vi "2013_01_05 Durability8 Main.vi"() -> ()   [LabVIEW 2011]
uses:
  MotorTypeDef.ctl
  <vilib>/DAQmx/write.llb/DAQmx Write (Counter Time 1Chan 1Samp).vi
  <vilib>/DAQmx/read.llb/DAQmx Read (Analog 1D Wfm NChan NSamp).vi
  <vilib>/Utility/TradDaqScaling.llb/Convert Thermistor Reading (waveform).vi
  <vilib>/DAQmx/miscellaneous.llb/DAQmx Fill In Error Info.vi
panel:
  in  "Y axis":u16(ring)=3 items=["RMS Current (A) 1"=1, "RMS Voltage (V) 1"=2, "RPM"=3, "Supply (V)"=4, "Torque (mNm)"=5, "Electrical Power (W)"=6, "Mechanical Power(W)"=7, "Motor Efficiency (%)"=8, "Source Current (A)"=10, "Supply Power (W)"=11, "ESC Efficiency (%)"=12, "Flow"=13, "Pressure Blue"=14, "Pressure Yellow"=15, "etc"=16]
  in  "X axis":u16(ring) items=["RMS Current (A) 1"=1, "RMS Voltage (V) 1"=2, "RPM"=3, "Supply (V)"=4, "Torque (mNm)"=5, "Electrical Power (W)"=6, "Mechanical Power(W)"=7, "Motor Efficiency (%)"=8, "Source Current (A)"=10, "Supply Power (W)"=11, "ESC Efficiency (%)"=12, "Flow"=13, "Pressure Blue"=14, "Pressure Yellow"=15, "Elapsed Time (s)"=0]
  out "XY Graph 2":cluster{"Array":dbl[], "Array":dbl[]}[](graph)
  out "Single Motor 2":waveform(dbl)[](graph)
  in  "Waveform":bool
  in  "Motor":dbl=1.0 min=1.0 max=8.0 step=1.0
  out "XY Graph":cluster{"Array":dbl[], "Array":dbl[]}[](graph)
  out "error out":errorcluster
  in  "File Path":path=path "Durability/.lvm"
  in  "Motor 8":T1 {"Power Input (W)" format="%.3g"; "Efficiency" format="%#_3g%%"; "Power Output (W)" format="%.3g"; "Torque (mNm)" format="%.3g"; "Elapsed Time" format="%<%H:%M:%S>t"; "Supply (V)" format="%.2f"; "RPM" scale=0.0..40000.0 scale format="%#_4p"}
  in  "Motor 7":T1 {"Power Input (W)" format="%.3g"; "Efficiency" format="%#_3g%%"; "Power Output (W)" format="%.3g"; "Torque (mNm)" format="%.3g"; "Elapsed Time" format="%<%H:%M:%S>t"; "Supply (V)" format="%.2f"; "RPM" scale=0.0..40000.0 scale format="%#_4p"}
  in  "Motor 6":T1 {"Power Input (W)" format="%.3g"; "Efficiency" format="%#_3g%%"; "Power Output (W)" format="%.3g"; "Torque (mNm)" format="%.3g"; "Elapsed Time" format="%<%H:%M:%S>t"; "Supply (V)" format="%.2f"; "RPM" scale=0.0..40000.0 scale format="%#_4p"}
  in  "Motor 5":T1 {"Power Input (W)" format="%.3g"; "Efficiency" format="%#_3g%%"; "Power Output (W)" format="%.3g"; "Torque (mNm)" format="%.3g"; "Elapsed Time" format="%<%H:%M:%S>t"; "Supply (V)" format="%.2f"; "RPM" scale=0.0..40000.0 scale format="%#_4p"}
  in  "Motor 4":T1 {"Power Input (W)" format="%.3g"; "Efficiency" format="%#_3g%%"; "Power Output (W)" format="%.3g"; "Torque (mNm)" format="%.3g"; "Elapsed Time" format="%<%H:%M:%S>t"; "Supply (V)" format="%.2f"; "RPM" scale=0.0..40000.0 scale format="%#_4p"}
  in  "Motor 3":T1 {"Power Input (W)" format="%.3g"; "Efficiency" format="%#_3g%%"; "Power Output (W)" format="%.3g"; "Torque (mNm)" format="%.3g"; "Elapsed Time" format="%<%H:%M:%S>t"; "Supply (V)" format="%.2f"; "RPM" scale=0.0..40000.0 scale format="%#_4p"}
  in  "Motor 2":T1 {"Power Input (W)" format="%.3g"; "Efficiency" format="%#_3g%%"; "Power Output (W)" format="%.3g"; "Torque (mNm)" format="%.3g"; "Elapsed Time" format="%<%H:%M:%S>t"; "Supply (V)" format="%.2f"; "RPM" scale=0.0..40000.0 scale format="%#_4p"}
  in  "Motor 1":T1 {"Power Input (W)" format="%.3g"; "Efficiency" format="%#_3g%%"; "Power Output (W)" format="%.3g"; "Torque (mNm)" format="%.3g"; "Elapsed Time" format="%<%H:%M:%S>t"; "Supply (V)" format="%.2f"; "RPM" scale=0.0..40000.0 scale format="%#_4p"}
  out "Motor Temp":dbl(slide) scale=65.0..110.0
  out "Tank Temp":dbl(slide) scale=65.0..110.0
  in  "Temp Probe\nOn Motor":dbl=1.0
  out "loop time (ms)":u32
  in  "stop":bool
  in  "Unlock PWM":bool=TRUE
  in  "PWM 2":dbl(slide)=100.0 min=0.0 max=100.0 step=5.0 scale=0.0..100.0
  in  "PWM 1":dbl(slide) min=0.0 max=100.0 step=5.0 scale=0.0..100.0
  # "Enable"
  # "Fail"
  # "Enable"
  # "Fail"
  # "Enable"
  # "Fail"
  # "Enable"
  # "Fail"
  # "Enable"
  # "Fail"
  # "Enable"
  # "Fail"
  # "Enable"
  # "Fail"
  # "Enable"
  # "Fail"
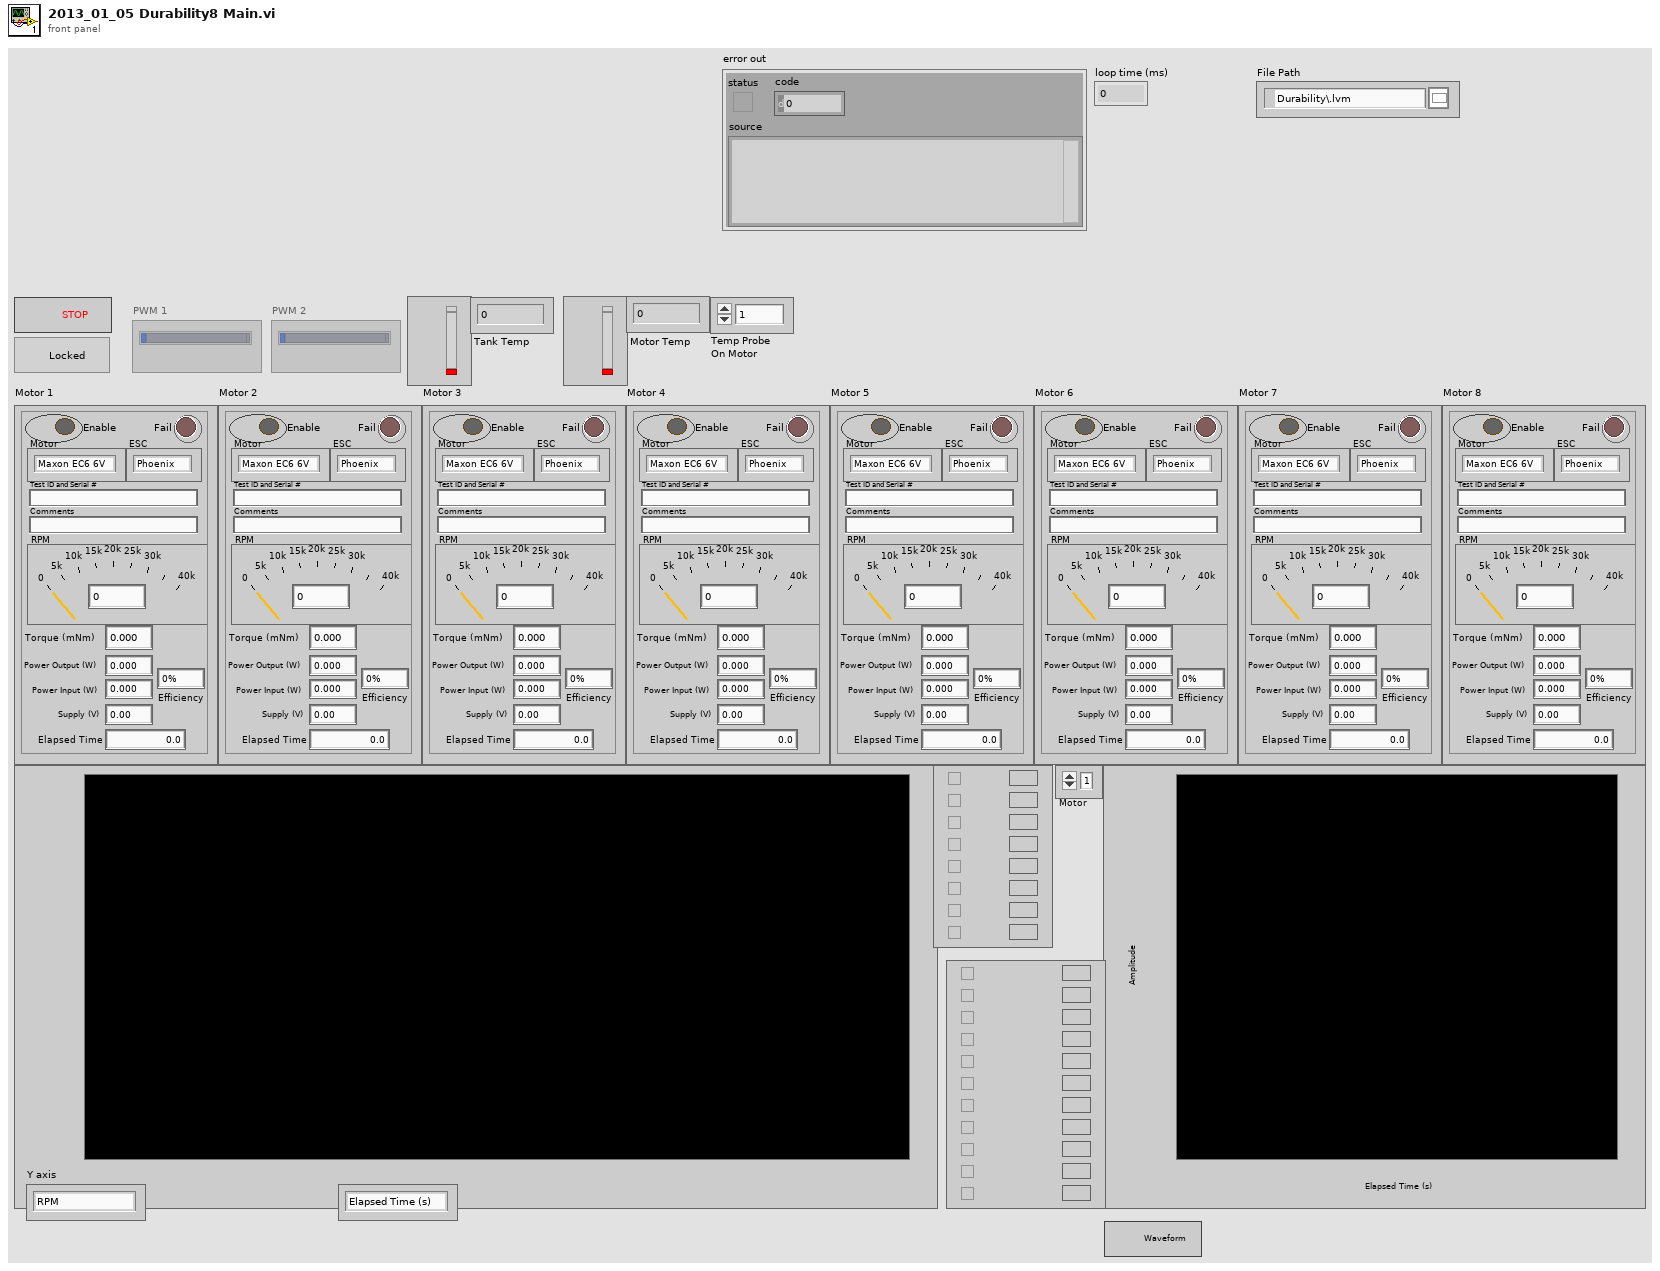
[diagram p1: front panel]
types:
  T1 = typedef "MotorTypeDef.ctl" = cluster{"Enabled":bool, "Fail":bool, "RPM":dbl, "Motor":enum16{"Maxon EC6 6V", "Maxon EC4 6V", "FH 0620 6V", "FH 0620 12V"}, "ESC":enum16{"Phoenix", "Maxon", "FH 1801"}, "Supply (V)":dbl, "Test ID and Serial #":string, "Comments":string, "Elapsed Time":dbl, "Counter":dbl, "Torque (mNm)":dbl, "Power Output (W)":dbl, "Efficiency":dbl, "Power Input (W)":dbl}
  T2 = enum8{"Enabled", "Disabled", "Disabled and Grayed Out"}
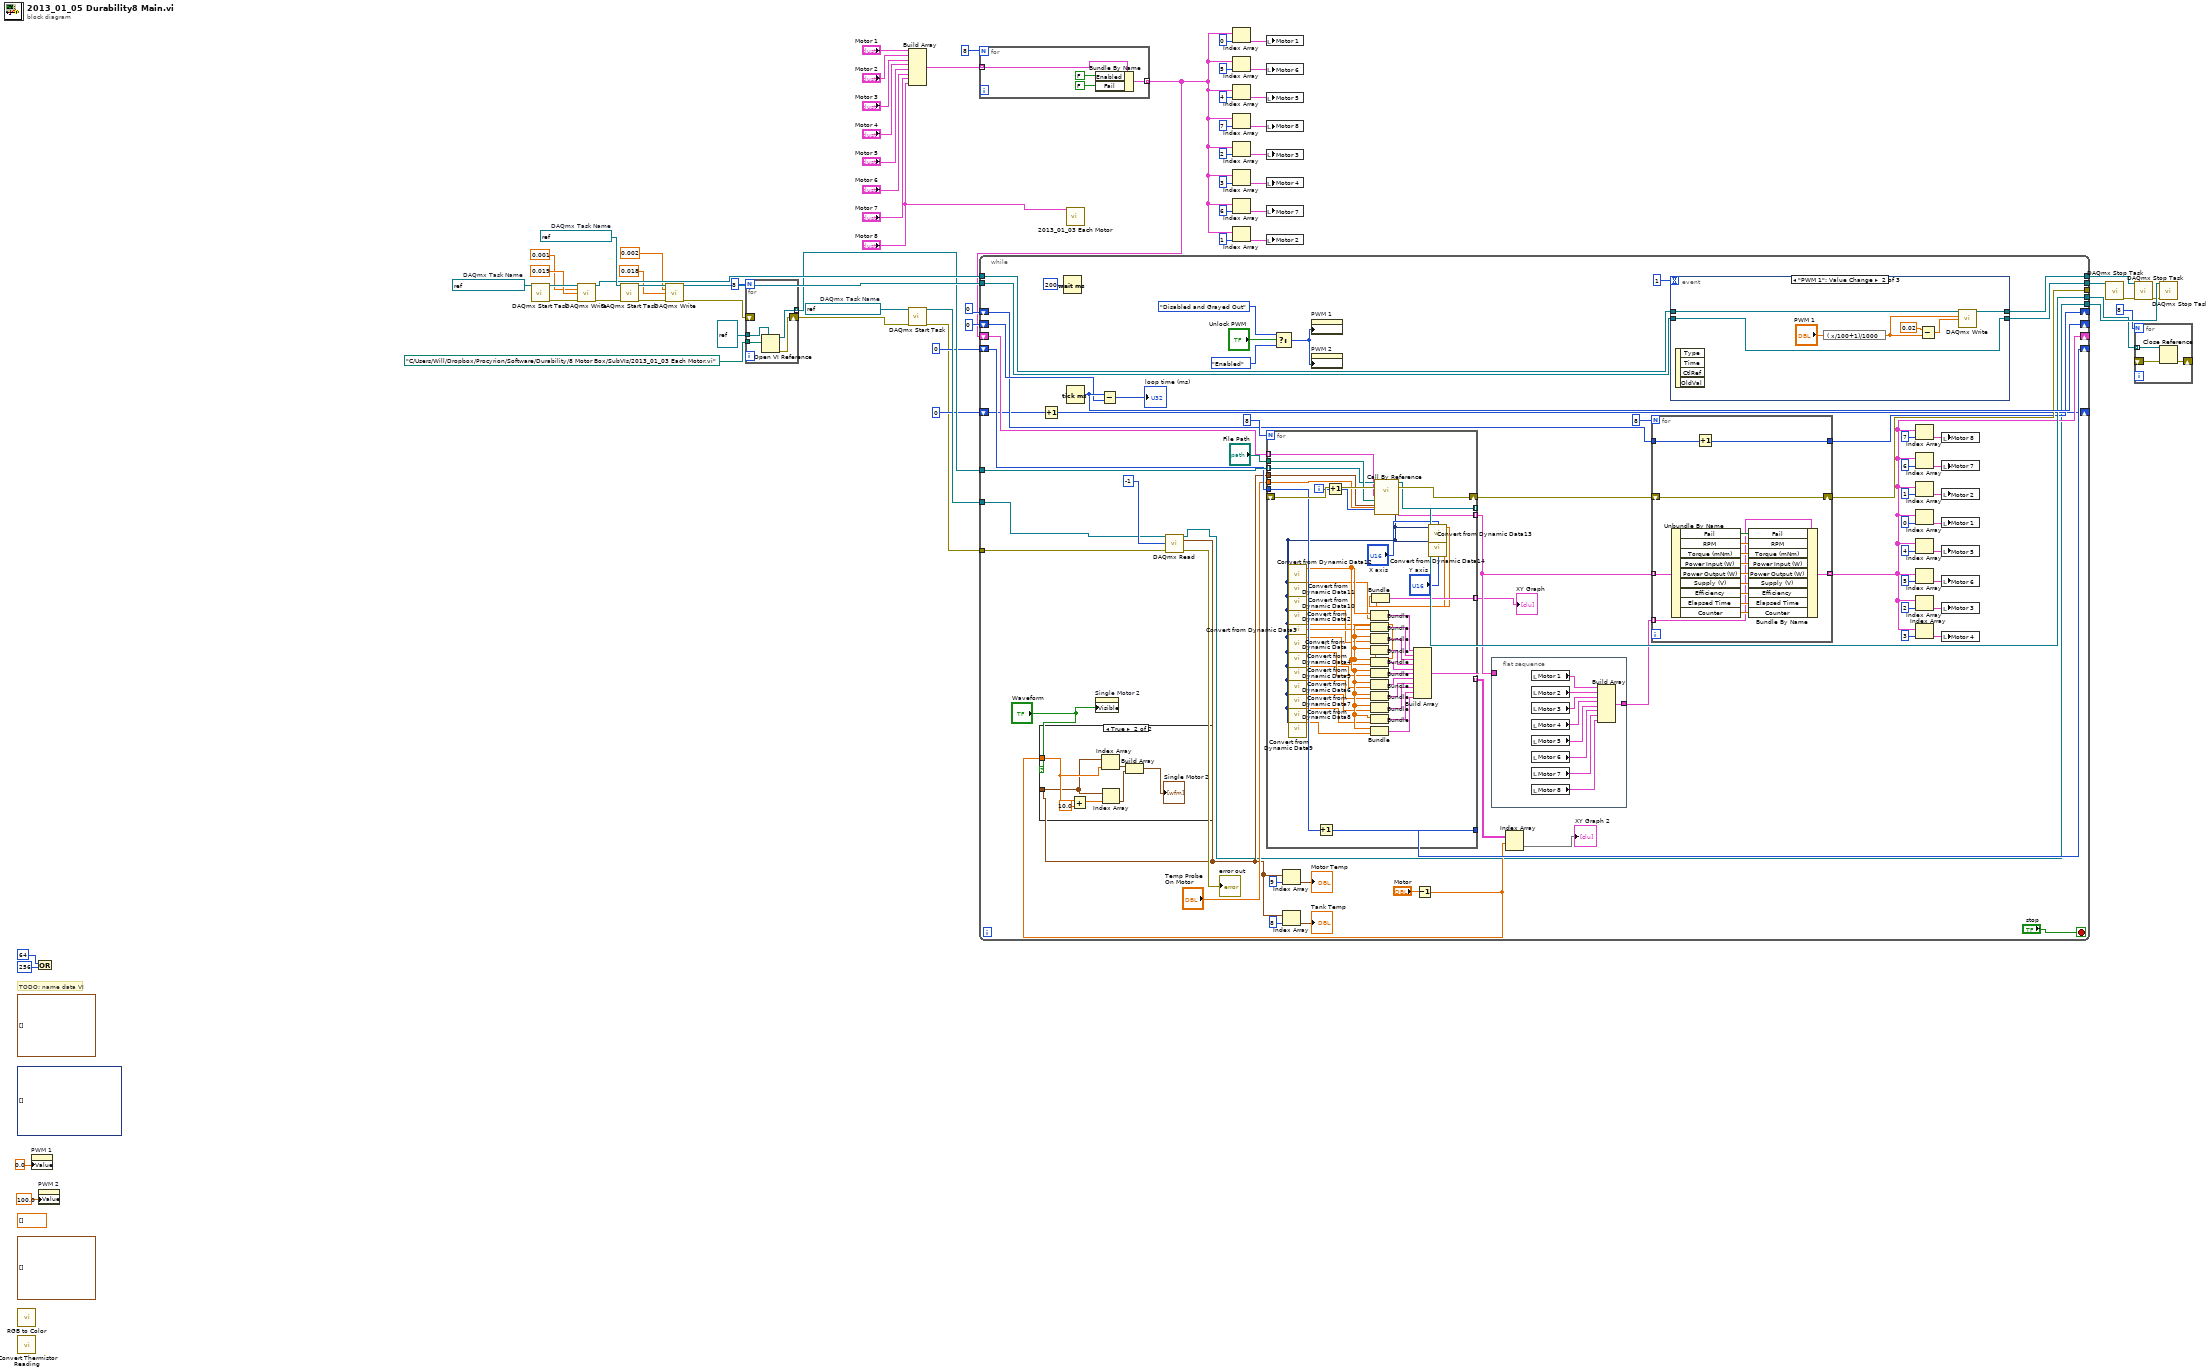
[diagram p0: block diagram]
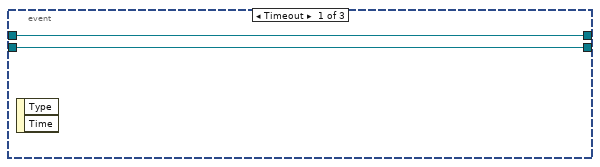
[diagram p3: hidden frame]
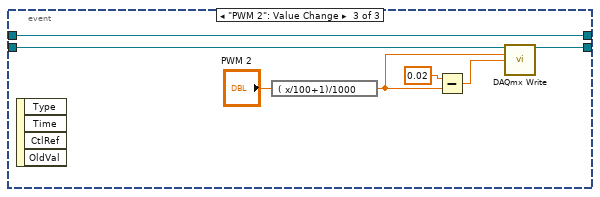
[diagram p4: hidden frame]
diagram:
  (unwired) dynamicdata[] []
  (unwired) dbl[] [] ("History Data")
  (unwired) waveform(dbl)[][] [] ("History Data")
  (unwired) waveform(dbl)[][] [] ("History Data")
  w60 = refnum<k21> "Durability8 PWM2"  # DAQmx Task Name
  w61 = refnum<k21> "Durability8 PWM1"  # DAQmx Task Name
  w64 = refnum<k21> "Durability8 Acquire"  # DAQmx Task Name
  # "TODO: name data VI"
  n1 = call <vilib>:"RGB to Color.vi"() -> ()  [unwired: 3 in, 1 out]
  n2 = call-poly <vilib>:"Convert Thermistor Reading.vi"() -> ()  [unwired: 7 in, 1 out]
  n3 = property on="PWM 1" class="Slide (strict)"("Value"=0.0 ("PWM 1")) -> ()  [unwired: 2 in, 2 out]
  n4 = Compound Arithmetic op=OR(64 ("options"), 256 ("options")) -> ()  [unwired: 1 out]
  n5 = property on="PWM 2" class="Slide (strict)"("Value"=100.0 ("PWM 2")) -> ()  [unwired: 2 in, 2 out]
  n6 = call <vilib>:"DAQmx Start Task.vi"("task/channels in"=w61) -> ("task out"=w57:refnum<k21>, "error out"=w55:errorcluster)  [unwired: 13 in]
  n7 = call-poly <vilib>:"DAQmx Write.vi"("task/channels in"=w57, "high time"=0.001 ("data"), "low time"=0.019 ("data"), "error in"=w55) -> ("task out"=w59:refnum<k21>, "error out"=w54:errorcluster)  [unwired: 9 in, 1 out]
  n8 = call <vilib>:"DAQmx Start Task.vi"("task/channels in"=w60, "error in"=w54) -> ("task out"=w56:refnum<k21>, "error out"=w53:errorcluster)  [unwired: 12 in]
  n9 = call-poly <vilib>:"DAQmx Write.vi"("task/channels in"=w56, "high time"=0.002 ("data"), "low time"=0.018 ("data"), "error in"=w53) -> ("task out"=w58:refnum<k21>, "error out"=w22:errorcluster)  [unwired: 9 in, 1 out]
  n10 = for {
    N: 8 -> [_]
    tunnel: path "C:/Users/Will/Dropbox/Procyrion/Software/Durability/8 Motor Box/SubVIs/2013_01_03 Each Motor.vi" -> [w68]
    tunnel: [w67] -> w38 mode=indexing
    tunnel: refnum<vi> refnum ("type specifier VI Refnum (for type only)") -> [w66]
    shift-right: [w65] -> w23
    shift-left: w22 -> [_]
    n11 = Open VI Reference(type specifier VI Refnum (for type only)=w66, vi path=w68) -> (vi reference=w67:refnum<vi>, error out=w65:errorcluster)  [unwired: 4 in]
  }
  n12 = Build Array("Motor 1", "Motor 2", "Motor 3", "Motor 4", "Motor 5", "Motor 6", "Motor 7", "Motor 8") -> (w19:T1[])
  n13 = call <vilib>:"DAQmx Start Task.vi"("task/channels in"=w64, "error in"=w23) -> ("task out"=w63:refnum<k21>, "error out"=w21:errorcluster)  [unwired: 12 in]
  n14 = for {
    N: 8 -> [_]
    tunnel: w19 -> [w72] mode=indexing
    tunnel: [w69] -> w2 mode=indexing
    n15 = Bundle By Name(cluster=w72, "Enabled"=FALSE, "Fail"=FALSE) -> (w69:T1)
  }
  n16 = while {
    tunnel: w63 -> [w73]
    tunnel: [w76] -> w62
    tunnel: w21 -> [w96]
    shift-right: [w132] -> _
    shift-left: u32 0 ("millisecond timer value") -> [w131]
    tunnel: w59 -> [w124]
    tunnel: w58 -> [w123]
    tunnel: [w122] -> w52
    tunnel: [w121] -> w45
    tunnel: w38 -> [w117]
    tunnel: [w116] -> w34
    shift-right: [w98] -> _
    shift-left: w2 -> [w97]
    tunnel: [w95] -> _
    shift-right: [w92] -> _
    shift-left: 0 ("for") -> [w93]
    shift-right: [w90] -> _
    shift-left: 0 ("for") -> [w91]
    shift-right: [w88] -> _
    shift-left: 0 ("for") -> [w89]
    stop <- "stop" stop-if-true
    n17 = Increment(x=w89) -> (x+1=w88:i32)
    n18 = Wait (ms)(milliseconds to wait=u32 200) -> ()  [unwired: 1 out]
    n19 = Tick Count (ms)() -> (millisecond timer value=w132:u32)
    n20 = property on="Single Motor 2" class="WFGraph (strict)"("Visible"="Waveform") -> ()  [unwired: 2 in, 2 out]
    n21 = Subtract(x=w132, y=w131) -> (x-y=→"loop time (ms)":u32)
    n22 = call-poly <vilib>:"DAQmx Read.vi"("task/channels in"=w73, "number of samples per channel"=-1, "error in"=w96) -> ("task out"=w76:refnum<k21>, "data"=w79:waveform(dbl)[], "error out"=→"error out":errorcluster)  [unwired: 10 in]
    n23 = for {
      N: 8 -> [_]
      tunnel: w79 -> [w222]
      tunnel: "File Path" -> [w223]
      tunnel: w117 -> [w220] mode=indexing
      shift-right: [w226] -> w94
      shift-left: _ -> [w225]
      tunnel: [w219] -> w116 mode=indexing
      tunnel: [w218] -> w86 mode=indexing
      tunnel: w97 -> [w184] mode=indexing
      tunnel: w93 -> [w217]
      tunnel: [w216] -> w92
      tunnel: "Temp Probe\nOn Motor" -> [w215]
      tunnel: [w214] -> w81 mode=indexing
      tunnel: [w201] -> w75 mode=indexing
      i -> [w224]
      n24 = Increment(x=w217) -> (x+1=w216:i32)
      n25 = Increment(x=w224) -> (x+1=w221:i32)
      n26 = call-by-ref "?"(reference=w220, error in=w225, "Temp On"=w215, "Motor #"=w221, "data"=w222, "File Path"=w223, "Motor Typedef"=w184) -> (reference out=w219:refnum<vi>, error out=w226:errorcluster, "Final Out"=w187:dynamicdata, "Motor Typedef Out"=w218:T1)  [unwired: 5 in]
      n27 = call "Convert from Dynamic Data12"("Dynamic Data Type"=w187) -> ("Array"=w202:dbl[])  [unwired: 3 in]
      n28 = call "Convert from Dynamic Data11"("Dynamic Data Type"=w187) -> ("Array"=w200:dbl[])  [unwired: 3 in]
      n29 = call "Convert from Dynamic Data10"("Dynamic Data Type"=w187) -> ("Array"=w199:dbl[])  [unwired: 3 in]
      n30 = call "Convert from Dynamic Data2"("Dynamic Data Type"=w187) -> ("Array"=w198:dbl[])  [unwired: 3 in]
      n31 = call "Convert from Dynamic Data3"("Dynamic Data Type"=w187) -> ("Array"=w197:dbl[])  [unwired: 3 in]
      n32 = call "Convert from Dynamic Data"("Dynamic Data Type"=w187) -> ("Array"=w196:dbl[])  [unwired: 3 in]
      n33 = call "Convert from Dynamic Data4"("Dynamic Data Type"=w187) -> ("Array"=w195:dbl[])  [unwired: 3 in]
      n34 = call "Convert from Dynamic Data5"("Dynamic Data Type"=w187) -> ("Array"=w194:dbl[])  [unwired: 3 in]
      n35 = call "Convert from Dynamic Data6"("Dynamic Data Type"=w187) -> ("Array"=w193:dbl[])  [unwired: 3 in]
      n36 = call "Convert from Dynamic Data7"("Dynamic Data Type"=w187) -> ("Array"=w192:dbl[])  [unwired: 3 in]
      n37 = call "Convert from Dynamic Data8"("Dynamic Data Type"=w187) -> ("Array"=w191:dbl[])  [unwired: 3 in]
      n38 = call "Convert from Dynamic Data9"("Dynamic Data Type"=w187) -> ("Array"=w190:dbl[])  [unwired: 3 in]
      n39 = Bundle("Array"=w202, "Array"=w200) -> (w203:cluster{"Array":dbl[], "Array":dbl[]})  [unwired: 1 in]
      n40 = Bundle("Array"=w202, "Array"=w199) -> (w204:cluster{"Array":dbl[], "Array":dbl[]})  [unwired: 1 in]
      n41 = Bundle("Array"=w202, "Array"=w198) -> (w205:cluster{"Array":dbl[], "Array":dbl[]})  [unwired: 1 in]
      n42 = Bundle("Array"=w202, "Array"=w197) -> (w206:cluster{"Array":dbl[], "Array":dbl[]})  [unwired: 1 in]
      n43 = Bundle("Array"=w202, "Array"=w196) -> (w207:cluster{"Array":dbl[], "Array":dbl[]})  [unwired: 1 in]
      n44 = Bundle("Array"=w202, "Array"=w195) -> (w208:cluster{"Array":dbl[], "Array":dbl[]})  [unwired: 1 in]
      n45 = Bundle("Array"=w202, "Array"=w194) -> (w209:cluster{"Array":dbl[], "Array":dbl[]})  [unwired: 1 in]
      n46 = Bundle("Array"=w202, "Array"=w193) -> (w210:cluster{"Array":dbl[], "Array":dbl[]})  [unwired: 1 in]
      n47 = Bundle("Array"=w202, "Array"=w192) -> (w212:cluster{"Array":dbl[], "Array":dbl[]})  [unwired: 1 in]
      n48 = Bundle("Array"=w202, "Array"=w191) -> (w211:cluster{"Array":dbl[], "Array":dbl[]})  [unwired: 1 in]
      n49 = Bundle("Array"=w202, "Array"=w190) -> (w213:cluster{"Array":dbl[], "Array":dbl[]})  [unwired: 1 in]
      n50 = Build Array(w203, w204, w205, w206, w207, w208, w209, w210, w212, w211, w213) -> (w201:cluster{"Array":dbl[], "Array":dbl[]}[])
      n51 = call "Convert from Dynamic Data13"("Dynamic Data Type"=w187, "Channel"="X axis") -> ("Array"=w186:dbl[])  [unwired: 2 in]
      n52 = call "Convert from Dynamic Data14"("Dynamic Data Type"=w187, "Channel"="Y axis") -> ("Array"=w185:dbl[])  [unwired: 2 in]
      n53 = Bundle("Array"=w186, "Array"=w185) -> (w214:cluster{"Array":dbl[], "Array":dbl[]})  [unwired: 1 in]
    }
    "XY Graph" <- w81
    n54 = Select(t=T2."Disabled and Grayed Out" ("Disabled"), s="Unlock PWM", f=T2."Enabled" ("Disabled")) -> (s? t:f=w136:T2)
    n55 = Index Array(array=w79, index=9) -> (element=→"Motor Temp":waveform(dbl))
    n56 = Index Array(array=w79, index=8) -> (element=→"Tank Temp":waveform(dbl))
    n57 = property on="PWM 1" class="Slide (strict)"("DisabledEnum"=w136) -> ()  [unwired: 2 in, 2 out]
    n58 = property on="PWM 2" class="Slide (strict)"("DisabledEnum"=w136) -> ()  [unwired: 2 in, 2 out]
    n59 = Decrement(x="Motor") -> (x-1=w78:dbl)
    n60 = case shown="True" "Waveform" {
      tunnel: w79 -> [_ w141]
      tunnel: w78 -> [_ w142]
      frame False {
      }
      frame True {
        n61 = Add(x=w142, y=10.0) -> (x+y=w140:dbl)
        n62 = Index Array(array=w141, index=w142) -> (element=w139:waveform(dbl))
        n63 = Index Array(array=w141, index=w140) -> (element=w138:waveform(dbl))
        n64 = Build Array(w139, w138) -> (→"Single Motor 2":waveform(dbl)[])
      }
    }
    n65 = flat-sequence {
      tunnel: [w145] -> w87
      tunnel: w86 -> [_]
      frame #0 {
        n66 = local read "Motor 1"() -> (w146:T1)
        n67 = local read "Motor 2"() -> (w147:T1)
        n68 = local read "Motor 3"() -> (w148:T1)
        n69 = local read "Motor 4"() -> (w149:T1)
        n70 = local read "Motor 5"() -> (w150:T1)
        n71 = local read "Motor 6"() -> (w151:T1)
        n72 = local read "Motor 7"() -> (w152:T1)
        n73 = local read "Motor 8"() -> (w144:T1)
        n74 = Build Array(w146, w147, w148, w149, w150, w151, w152, w144) -> (w145:T1[])
      }
    }
    n75 = Index Array(array=w75, index (row)=w78) -> (element=→"XY Graph 2":cluster{"Array":dbl[], "Array":dbl[]}[])  [unwired: 1 in]
    n76 = for {
      N: 8 -> [_]
      tunnel: w87 -> [w158] mode=indexing
      tunnel: [w157] -> w98 mode=indexing
      tunnel: w86 -> [w156] mode=indexing
      shift-right: [w155] -> w95
      shift-left: w94 -> [w155]
      tunnel: [w153] -> w90
      tunnel: w91 -> [w154]
      n77 = Unbundle By Name(w156) -> ("Fail"=w167:bool, "RPM"=w166:dbl, "Torque (mNm)"=w165:dbl, "Power Input (W)"=w164:dbl, "Power Output (W)"=w163:dbl, "Supply (V)"=w162:dbl, "Efficiency"=w161:dbl, "Elapsed Time"=w160:dbl, "Counter"=w159:dbl)
      n78 = Increment(x=w154) -> (x+1=w153:i32)
      n79 = Bundle By Name(cluster=w158, "Fail"=w167, "RPM"=w166, "Torque (mNm)"=w165, "Power Input (W)"=w164, "Power Output (W)"=w163, "Supply (V)"=w162, "Efficiency"=w161, "Elapsed Time"=w160, "Counter"=w159) -> (w157:T1)
    }
    n80 = event shown="[1] \"PWM 1\": Value Change" {
      selector: _ -> [_ _ _]
      dyn-events: _ -> [_ _ _]
      timeout: 1 -> [_ _ _]
      tunnel: w124 -> [w169 w172 w178]
      tunnel: w123 -> [w168 w170 w177]
      tunnel: [w169 w171 w178] -> w122
      tunnel: [w168 w170 w179] -> w121
      event Timeout {
        n81 = event-data() -> ()  [unwired: 1 in, 2 out]
      }
      event "PWM 1": Value Change {
        n82 = event-data() -> ()  [unwired: 1 in, 4 out]
        n83 = expression code="( x/100+1)/1000"("PWM 1") -> (w173:dbl)
        n84 = Subtract(x=0.02 ("y"), y=w173) -> (x-y=w174:dbl)
        n85 = call-poly <vilib>:"DAQmx Write.vi"("task/channels in"=w172, "high time"=w173, "low time"=w174) -> ("task out"=w171:refnum<k21>)  [unwired: 10 in, 2 out]
      }
      event "PWM 2": Value Change {
        n86 = event-data() -> ()  [unwired: 1 in, 4 out]
        n87 = expression code="( x/100+1)/1000"("PWM 2") -> (w183:dbl)
        n88 = Subtract(x=0.02, y=w183) -> (x-y=w181:dbl)
        n89 = call-poly <vilib>:"DAQmx Write.vi"("task/channels in"=w177, "high time"=w183, "low time"=w181) -> ("task out"=w179:refnum<k21>)  [unwired: 10 in, 2 out]
      }
    }
    n90 = Index Array(array=w98, index=7) -> (element=w105:T1)
    n91 = Index Array(array=w98, index=6) -> (element=w104:T1)
    n92 = Index Array(array=w98, index=1) -> (element=w99:T1)
    n93 = Index Array(array=w98, index=0) -> (element=w114:T1)
    n94 = Index Array(array=w98, index=4) -> (element=w102:T1)
    n95 = Index Array(array=w98, index=5) -> (element=w103:T1)
    n96 = Index Array(array=w98, index=2) -> (element=w100:T1)
    n97 = Index Array(array=w98, index=3) -> (element=w101:T1)
    n98 = local write "Motor 8"(w105) -> ()
    n99 = local write "Motor 7"(w104) -> ()
    n100 = local write "Motor 2"(w99) -> ()
    n101 = local write "Motor 1"(w114) -> ()
    n102 = local write "Motor 5"(w102) -> ()
    n103 = local write "Motor 6"(w103) -> ()
    n104 = local write "Motor 3"(w100) -> ()
    n105 = local write "Motor 4"(w101) -> ()
  }
  n106 = call "2013_01_03 Each Motor.vi"("Motor Typedef"="Motor 8") -> ()  [unwired: 9 in, 2 out]
  n107 = Index Array(array=w2, index=0) -> (element=w18:T1)
  n108 = Index Array(array=w2, index=5) -> (element=w7:T1)
  n109 = Index Array(array=w2, index=4) -> (element=w6:T1)
  n110 = Index Array(array=w2, index=7) -> (element=w9:T1)
  n111 = Index Array(array=w2, index=2) -> (element=w4:T1)
  n112 = Index Array(array=w2, index=3) -> (element=w5:T1)
  n113 = Index Array(array=w2, index=6) -> (element=w8:T1)
  n114 = Index Array(array=w2, index=1) -> (element=w3:T1)
  n115 = local write "Motor 1"(w18) -> ()
  n116 = local write "Motor 6"(w7) -> ()
  n117 = local write "Motor 5"(w6) -> ()
  n118 = local write "Motor 8"(w9) -> ()
  n119 = local write "Motor 3"(w4) -> ()
  n120 = local write "Motor 4"(w5) -> ()
  n121 = local write "Motor 7"(w8) -> ()
  n122 = local write "Motor 2"(w3) -> ()
  n123 = call <vilib>:"DAQmx Stop Task.vi"("task/channels in"=w45) -> ("error out"=w51:errorcluster)  [unwired: 13 in, 1 out]
  n124 = call <vilib>:"DAQmx Stop Task.vi"("task/channels in"=w52, "error in"=w51) -> ("error out"=w50:errorcluster)  [unwired: 12 in, 1 out]
  n125 = for {
    N: 8 -> [_]
    shift-right: [w229] -> _
    shift-left: _ -> [w227]
    tunnel: w34 -> [w228] mode=indexing
    n126 = Close Reference(reference=w228, error in (no error)=w227) -> (error out=w229:errorcluster)
  }
  n127 = call <vilib>:"DAQmx Stop Task.vi"("task/channels in"=w62, "error in"=w50) -> ()  [unwired: 12 in, 2 out]
